vi "GetMyIPAddress.vi"(2 "Port":u32=5000, 3 "Format":T1(ring)) -> (0 "URI":string="http://192.168.1.8", 1 "Good?":bool)   [LabVIEW 2016]
doc: "Returns your IP address"
uses:
  _ROSDefinition.vi
panel:
  out "Available addresses":string[](array[string])
  out "IP Address":string
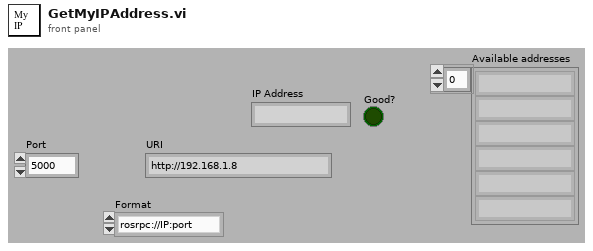
[diagram p1: front panel]
types:
  T1 = enum16{"rosrpc://IP:port", "http://IP:port", "http://IP", "IP:port", "IP only"}
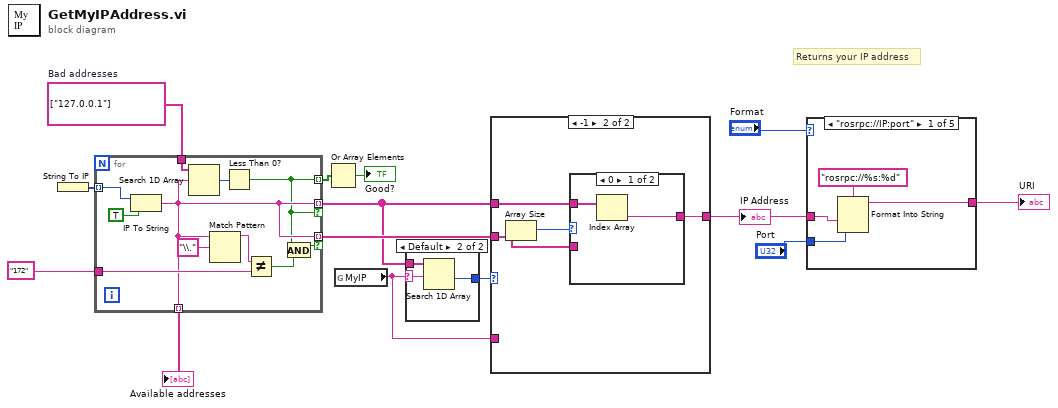
[diagram p0: block diagram]
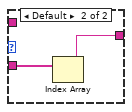
[diagram p3: hidden frame]
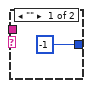
[diagram p4: hidden frame]
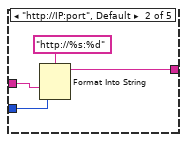
[diagram p5: hidden frame]
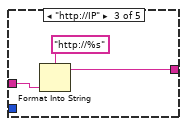
[diagram p6: hidden frame]
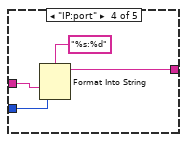
[diagram p7: hidden frame]
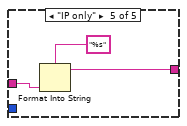
[diagram p8: hidden frame]
diagram:
  w9 = string[] ["127.0.0.1"]  # Bad addresses
  # "Returns your IP address"
  n1 = String To IP() -> (0:w10:u32[])  [unwired: 1 in]
  n2 = for {
    tunnel: [w18] -> w3 mode=indexing if=w16
    tunnel: w10 -> [w25] mode=indexing
    tunnel: w9 -> [w23]
    tunnel: [w16] -> w8 mode=indexing
    tunnel: [w18] -> w7 mode=indexing
    tunnel: "172" ("IP Address") -> [w19]
    tunnel: [w18] -> w4 mode=indexing if=w15
    n3 = IP To String(1:TRUE ("dot notation? (F)"), 2:w25) -> (0:w18:string)
    n4 = Search 1D Array(1D array=w23, element=w18) -> (index of element=w22:i32)  [unwired: 1 in]
    n5 = Match Pattern(string=w18, regular expression="\\.") -> (before substring=w20:string)  [unwired: 1 in, 3 out]
    n6 = Less Than 0?(x=w22) -> (x < 0?=w16:bool)
    n7 = Not Equal?(x=w20, y=w19) -> (x != y?=w17:bool)
    n8 = And(x=w16, y=w17) -> (x .and. y?=w15:bool)
  }
  "Available addresses" <- w7
  n9 = Or Array Elements(Boolean array=w8) -> (logical OR=→"Good?":bool)
  n10 = global read "_ROSDefinition.vi" "MyIP"() -> (w1:string)
  n11 = case shown="Default" w1 {
    selector: w1 -> [_ w28]
    tunnel: w3 -> [_ w29]
    tunnel: [-1 ("index of element") w27] -> w2
    frame "" {
    }
    frame Default {
      n12 = Search 1D Array(1D array=w29, element=w28) -> (index of element=w27:i32)  [unwired: 1 in]
    }
  }
  n13 = case shown="-1" w2 {
    tunnel: [w30 w34] -> w11
    tunnel: w4 -> [_ w32]
    tunnel: w3 -> [_ w31]
    tunnel: w1 -> [w30 _]
    frame Default {
    }
    frame -1 {
      n14 = Array Size(array=w32) -> (size(s)=w33:i32)
      n15 = case shown="0" w33 {
        tunnel: w31 -> [w36 _]
        tunnel: [w35 w37] -> w34
        tunnel: w32 -> [_ w38]
        frame 0 {
          n16 = Index Array(array=w36) -> (element=w35:string)  [unwired: 1 in]
        }
        frame Default {
          n17 = Index Array(array=w38) -> (element=w37:string)  [unwired: 1 in]
        }
      }
    }
  }
  "IP Address" <- w11
  n18 = case shown="\"rosrpc://IP:port\"" "Format" {
    tunnel: w11 -> [w41 w45 w48 w52 w55]
    tunnel: "Port" -> [w40 w44 _ w50 _]
    tunnel: [w39 w43 w47 w51 w54] -> w14
    frame "rosrpc://IP:port" {
      n19 = Format Into String(format string="rosrpc://%s:%d", w41, w40) -> (resulting string=w39:string)  [unwired: 2 in, 1 out]
    }
    frame "http://IP:port", Default {
      n20 = Format Into String(format string="http://%s:%d", w45, w44) -> (resulting string=w43:string)  [unwired: 2 in, 1 out]
    }
    frame "http://IP" {
      n21 = Format Into String(format string="http://%s", w48) -> (resulting string=w47:string)  [unwired: 2 in, 1 out]
    }
    frame "IP:port" {
      n22 = Format Into String(format string="%s:%d", w52, w50) -> (resulting string=w51:string)  [unwired: 2 in, 1 out]
    }
    frame "IP only" {
      n23 = Format Into String(format string="%s", w55) -> (resulting string=w54:string)  [unwired: 2 in, 1 out]
    }
  }
  "URI" <- w14
